vi "DIAdem Response Handler.vi"(6 "Wait? (T)":bool, 8 "error in (no error)":errorcluster, 10 "Response String (\"\")":string, 11 "Response Queue Name (\"\")":string) -> (0 "error out":errorcluster, 2 "Response String":string)   [LabVIEW 2011]
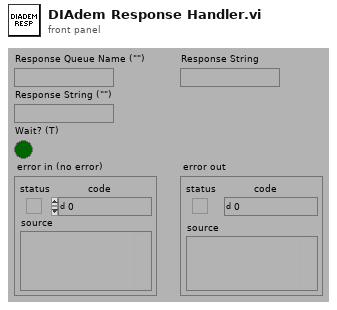
[diagram p1: front panel]
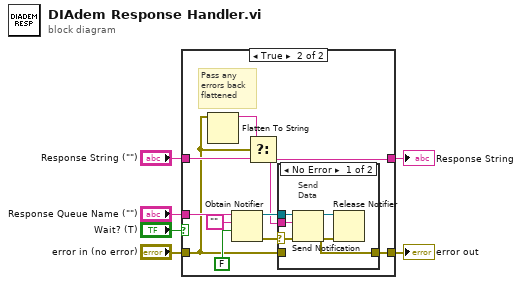
[diagram p0: block diagram]
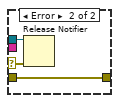
[diagram p3: hidden frame]
diagram:
  n1 = case shown="True" "Wait? (T)" {
    tunnel: "Response Queue Name (\"\")" -> [_ w13]
    tunnel: "Response String (\"\")" -> [w7 w12]
    tunnel: "error in (no error)" -> [w8 w11]
    tunnel: [w8 w10] -> w3
    tunnel: [w7 w9] -> w1
    frame False {
    }
    frame True {
      # "Pass any\nerrors back\nflattened"
      n2 = Flatten To String(anything=w11) -> (data string=w16:string)  [unwired: 1 in, 4 out]
      n3 = Obtain Notifier(name (unnamed)=w13, notification data type="", create if not found? (T)=FALSE) -> (notifier out=w14:refnum<notifier>, error out=w15:errorcluster)  [unwired: 1 in, 1 out]
      n4 = Select(t=w16, s=w11, f=w12) -> (s? t:f=w9:string)
      n5 = case shown="No Error" w15 {
        selector: w15 -> [w21 w24]
        tunnel: w9 -> [w23 _]
        tunnel: [w19 w26] -> w10
        tunnel: w14 -> [w22 w25]
        tunnel: w11 -> [_ w26]
        frame No Error {
          # "Send\nData"
          n6 = Send Notification(notification=w23, notifier=w22, error in (no error)=w21) -> (notifier out=w20:refnum<notifier>, error out=w19:errorcluster)
          n7 = Release Notifier(notifier=w20, error in (no error)=w19) -> ()  [unwired: 4 out]
        }
        frame Error {
          n8 = Release Notifier(notifier=w25, error in (no error)=w24) -> ()  [unwired: 4 out]
        }
      }
    }
  }
  "error out" <- w3
  "Response String" <- w1
